vi "THETA_3_4.vi"(8 "error in (no error)":errorcluster, 11 "reference in":refnum<class "Manipulator.lvclass">) -> (0 "error out":errorcluster, 3 "reference out":refnum<class "Manipulator.lvclass">)   [LabVIEW 2014, in "Manipulator.lvclass"]
uses:
  Manipulator.lvclass
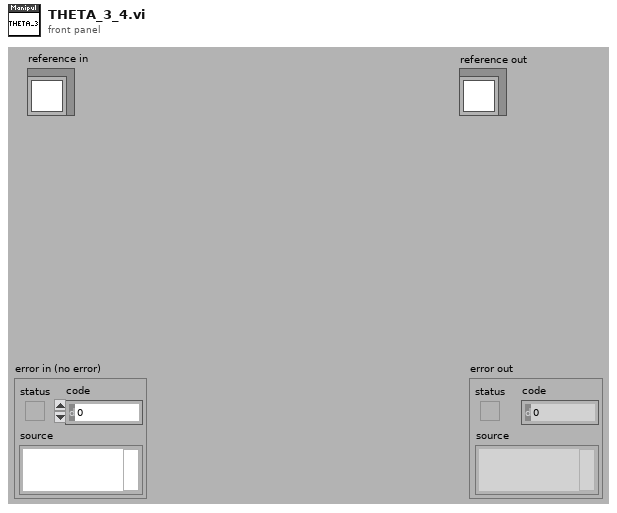
[diagram p1: front panel]
types:
  T1 = typedef "Manipulator.lvclass/ObjectAttributes.ctl" = cluster{"Coordinates":cluster{"X":dbl, "Y":dbl, "Z":dbl}, "Angles":cluster{"THETA_1":dbl, "THETA_2":dbl, "THETA_3":dbl, "THETA_4":dbl, "THETA_5":dbl, "THETA_6":dbl, "THETA_7":dbl, "THETA_8":dbl, "THETA_9":dbl, "THETA_10":dbl}, "Lengths":cluster{"a":dbl, "b":dbl, "c":dbl, "d":dbl, "e":dbl}}
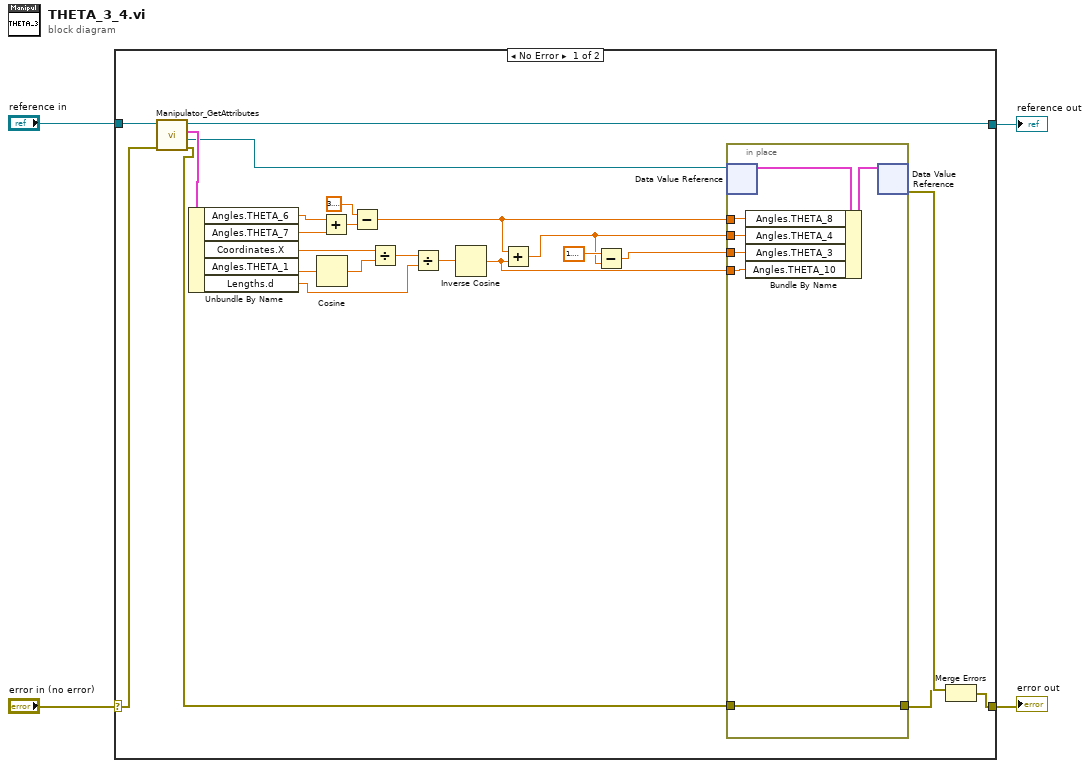
[diagram p0: block diagram]
diagram:
  n1 = case shown="No Error" "error in (no error)" {
    selector: "error in (no error)" -> [w27 w37]
    tunnel: [w23 w37] -> w3
    tunnel: [w24 w36] -> w1
    tunnel: "reference in" -> [w28 w36]
    frame No Error {
      n2 = call "Manipulator_GetAttributes.vi"("error in (no error)"=w27, "reference in"=w28) -> ("error out"=w21:errorcluster, "DataRef"=w22:refnum<data-value>, "Data"=w26:T1, "reference out"=w24:refnum<class "Manipulator.lvclass">)  [unwired: 6 in]
      n3 = Unbundle By Name(w26) -> ("Angles.THETA_6"=w19:dbl, "Angles.THETA_7"=w18:dbl, "Coordinates.X"=w14:dbl, "Angles.THETA_1"=w15:dbl, "Lengths.d"=w11:dbl)
      n4 = Cosine(x=w15) -> (cos(x)=w13:dbl)
      n5 = Add(x=w19, y=w18) -> (x+y=w16:dbl)
      n6 = Subtract(x=3.141592653589793, y=w16) -> (x-y=w9:dbl)
      n7 = Divide(x=w14, y=w13) -> (x/y=w12:dbl)
      n8 = Divide(x=w12, y=w11) -> (x/y=w10:dbl)
      n9 = Inverse Cosine(1:w10) -> (0:w5:dbl)
      n10 = Add(x=w9, y=w5) -> (x+y=w7:dbl)
      n11 = Subtract(x=1.5707963267948966, y=w7) -> (x-y=w6:dbl)
      n12 = in-place {
        in-place-border: w21 -> [w34]
        in-place-border: [w34] -> w20
        in-place-border: w9 -> [w32]
        in-place-border: w7 -> [w31]
        in-place-border: w6 -> [w30]
        in-place-border: w5 -> [w29]
        n13 = in-place-dvr #1(w22) -> (w33:T1)  [unwired: 1 out]
        n14 = Bundle By Name(cluster=w33, "Angles.THETA_8"=w32, "Angles.THETA_4"=w31, "Angles.THETA_3"=w30, "Angles.THETA_10"=w29) -> (w35:T1)
        n15 = in-place-dvr #1(w35) -> (w25:errorcluster)  [unwired: 1 out]
      }
      n16 = Merge Errors(w25, w20) -> (w23:errorcluster)
    }
    frame Error {
    }
  }
  "error out" <- w3
  "reference out" <- w1
